vi "PH_Cont-601k_PSU.Action Charge.vi"(0 "VI in":refnum<vi>, 5 "error in (no error)":errorcluster) -> (14 "VI out":refnum<vi>, 19 "error out":errorcluster)   [LabVIEW 2014, in "PH_Cont-601k_PSU.lvlib"]
uses:
  PH_Cont-601k_PSU.lvlib
  PH_Cont-601k_PSU.Readyness Device.ctl
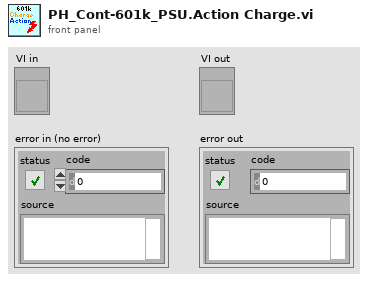
[diagram p1: front panel]
types:
  T1 = typedef "PH_Cont-601k_PSU.lvlib/PH_Cont-601k_PSU.Readyness Device.ctl" = enum32{"OFF", "CONNECTING", "CONNECTED", "OPERATING", "EOC", "ERROR"}
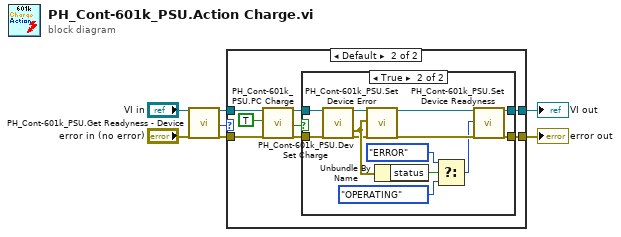
[diagram p0: block diagram]
diagram:
  n1 = call "PH_Cont-601k_PSU.Get Readyness - Device.vi"("VI in"="VI in", "error in (no error)"="error in (no error)") -> ("VI out"=w6:refnum<vi>, "Readyness - Device"=w7:T1, "error out"=w4:errorcluster)  [unwired: 15 in]
  n2 = case shown="Default" w7 {
    tunnel: [w9 w17] -> w2
    tunnel: [w8 w16] -> w3
    tunnel: w4 -> [w8 w15]
    tunnel: w6 -> [w9 w14]
    frame "OFF" {
    }
    frame Default {
      n3 = call "PH_Cont-601k_PSU.PC Charge.vi"("VI in"=w14, "Charge"=TRUE ("Configuration changed?"), "error in (no error)"=w15) -> ("VI out"=w13:refnum<vi>, "\"Charge\" changed"=w11:bool, "error out"=w12:errorcluster)  [unwired: 14 in]
      n4 = case shown="True" w11 {
        tunnel: w13 -> [w19 w32]
        tunnel: w12 -> [w18 w31]
        tunnel: [w19 w21] -> w17
        tunnel: [w18 w20] -> w16
        frame False {
        }
        frame True {
          n5 = call "PH_Cont-601k_PSU.Dev Set Charge.vi"("VI in"=w32, "error in (no error)"=w31) -> ("VI out"=w23:refnum<vi>, "Device Error out"=w24:errorcluster, "error out"=w22:errorcluster)  [unwired: 15 in]
          n6 = call "PH_Cont-601k_PSU.Set Device Error.vi"("VI in"=w23, "Device Error"=w24, "error in (no error)"=w22) -> ("VI out"=w29:refnum<vi>, "error out"=w30:errorcluster)  [unwired: 15 in]
          n7 = Unbundle By Name(w24) -> ("status"=w26:bool)
          n8 = Select(t=PH_Cont-601k_PSU.Readyness_Device."ERROR" ("Readyness.Device"), s=w26, f=PH_Cont-601k_PSU.Readyness_Device."OPERATING" ("Readyness Device to set")) -> (s? t:f=w28:T1)
          n9 = call "PH_Cont-601k_PSU.Set Device Readyness.vi"("VI in"=w29, "Readyness Device to set"=w28, "error in (no error)"=w30) -> ("VI out"=w21:refnum<vi>, "error out"=w20:errorcluster)  [unwired: 15 in]
        }
      }
    }
  }
  "error out" <- w3
  "VI out" <- w2
